vi "move.vi"   [LabVIEW 2018]
uses:
  User32.dll
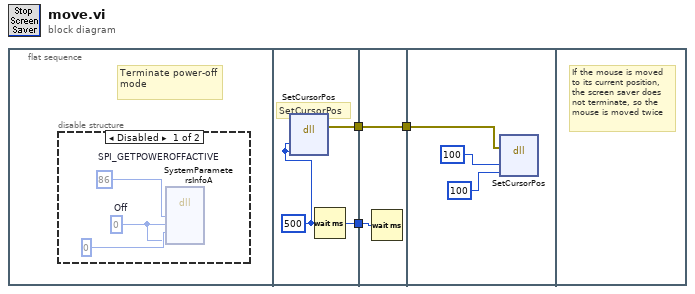
[diagram p0: block diagram]
diagram:
  n1 = flat-sequence {
    tunnel: [w8] -> w3
    tunnel: [w7] -> w1
    tunnel: w3 -> [w11]
    tunnel: [w11] -> w2
    tunnel: w1 -> [w10]
    tunnel: w2 -> [w12]
    frame #0 {
      # "Terminate power-off mode"
      n2 = disable-structure shown="Disabled" {
        frame Disabled {
          w4 = u32 0  # Off
          w6 = u32 86  # SPI_GETPOWEROFFACTIVE
          n3 = dll-call lib="User32.dll" fn="SystemParametersInfoA"("uiAction"=w6, "uiParam"=w4, "pvParam"=0, "fWinIni"=w4) -> ()  [unwired: 8 in, 2 out]
        }
        frame Enabled {
        }
      }
    }
    frame #1 {
      w9 = u32 500 ("milliseconds to wait")
      # "SetCursorPos"
      n4 = dll-call lib="User32.dll" fn="SetCursorPos"(w9, w9) -> (error out=w8:errorcluster)  [unwired: 6 in, 1 out]
      n5 = Wait (ms)(milliseconds to wait=w9) -> (millisecond timer value=w7:u32)
    }
    frame #2 {
      n6 = Wait (ms)(milliseconds to wait=w10) -> ()  [unwired: 1 out]
    }
    frame #3 {
      n7 = dll-call lib="User32.dll" fn="SetCursorPos" label="Move mouse to new pos"(error in=w12, "dx"=100, "dy"=100 ("dx")) -> ()  [unwired: 5 in, 2 out]
    }
    frame #4 {
      # "If the mouse is moved to its current position, the screen saver does not terminate, so the mouse is moved twice"
    }
  }
